vi "main.vi"() -> ()   [LabVIEW 2018]
panel:
  in  "stop":bool
  out "Numeric":i32
  out "A0":bool
  out "A1":bool
  out "A2":bool
  out "A4":bool
  in  "Count":bool
  in  "Load":bool
  in  "I0":bool
  in  "I1":bool
  in  "I2":bool
  in  "I3":bool
  out "Finish":bool
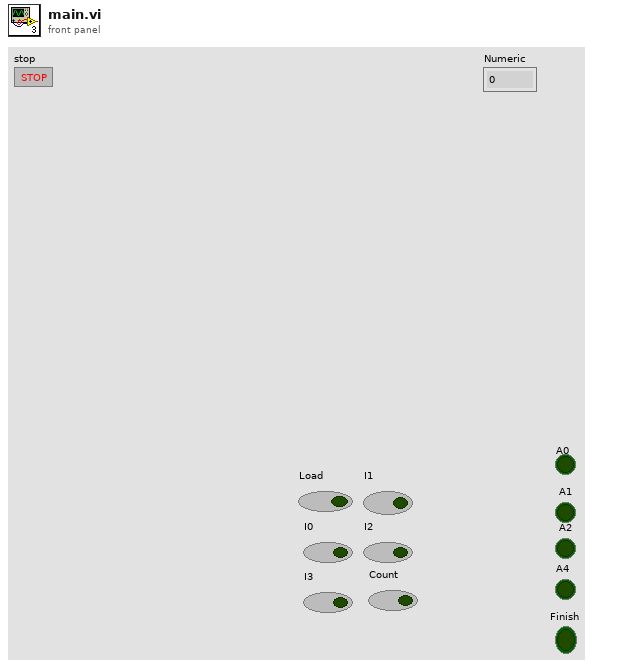
[diagram p1: front panel]
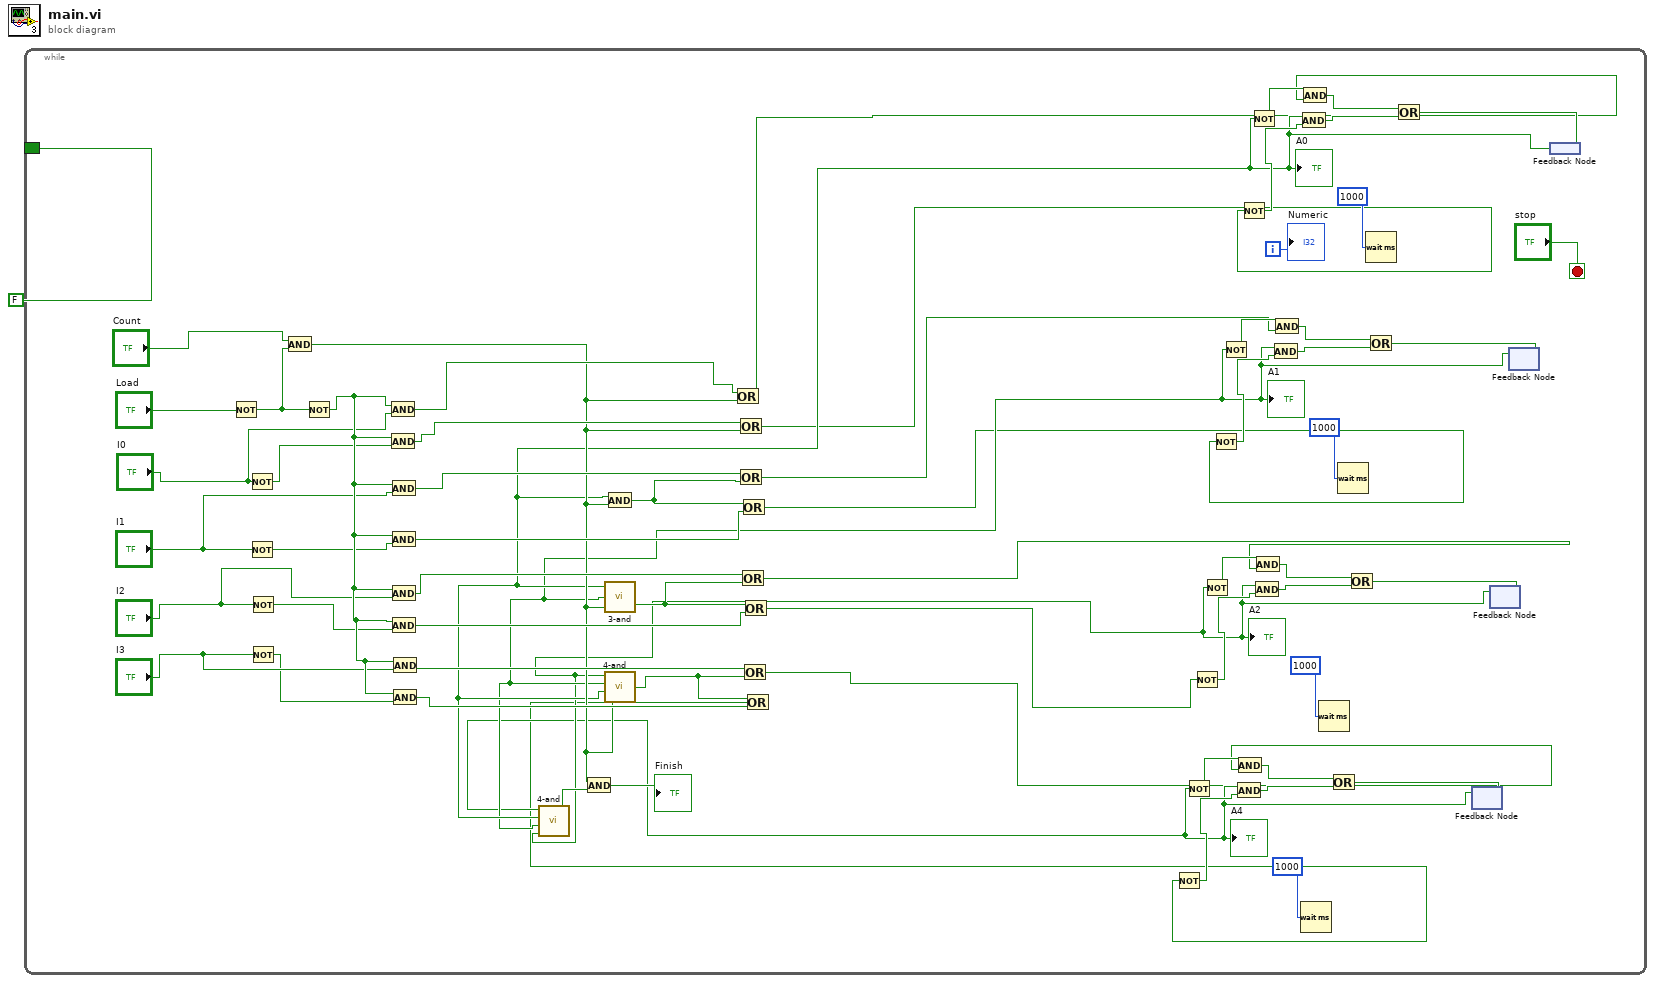
[diagram p0: block diagram]
diagram:
  n1 = while {
    border: FALSE -> [_]
    i -> [w63]
    stop <- "stop" stop-if-true
    n2 = Not(x="Load") -> (.not. x?=w37:bool)
    n3 = Not(x="I0") -> (.not. x?=w34:bool)
    n4 = Not(x="I1") -> (.not. x?=w32:bool)
    n5 = Not(x="I2") -> (.not. x?=w30:bool)
    n6 = Not(x="I3") -> (.not. x?=w28:bool)
    n7 = And(x="Count", y=w37) -> (x .and. y?=w16:bool)
    n8 = Not(x=w37) -> (.not. x?=w36:bool)
    n9 = And(x=w36, y="I0") -> (x .and. y?=w26:bool)
    n10 = And(x=w36, y=w34) -> (x .and. y?=w25:bool)
    n11 = And(x=w36, y="I1") -> (x .and. y?=w24:bool)
    n12 = And(x=w36, y=w32) -> (x .and. y?=w23:bool)
    n13 = And(x=w36, y="I2") -> (x .and. y?=w22:bool)
    n14 = And(x=w36, y=w30) -> (x .and. y?=w21:bool)
    n15 = And(x=w36, y="I3") -> (x .and. y?=w20:bool)
    n16 = And(x=w36, y=w28) -> (x .and. y?=w19:bool)
    n17 = Or(x=w26, y=w16) -> (x .or. y?=w12:bool)
    n18 = Or(x=w25, y=w16) -> (x .or. y?=w11:bool)
    n19 = Not(x=w11) -> (.not. x?=w58:bool)
    n20 = Wait (ms)(milliseconds to wait=u32 1000) -> ()  [unwired: 1 out]
    n21 = Wait (ms)(milliseconds to wait=u32 1000) -> ()  [unwired: 1 out]
    n22 = Wait (ms)(milliseconds to wait=u32 1000) -> ()  [unwired: 1 out]
    n23 = Wait (ms)(milliseconds to wait=u32 1000) -> ()  [unwired: 1 out]
    n24 = feedback #1() -> (w4:bool)  [unwired: 1 in]
    "A4" <- w4
    n25 = Not(x=w4) -> (.not. x?=w41:bool)
    n26 = feedback #2() -> (w7:bool)  [unwired: 1 in]
    "A2" <- w7
    n27 = Not(x=w7) -> (.not. x?=w47:bool)
    n28 = feedback #3() -> (w10:bool)  [unwired: 1 in]
    "A1" <- w10
    n29 = Not(x=w10) -> (.not. x?=w53:bool)
    n30 = feedback #4() -> (w13:bool)
    "A0" <- w13
    n31 = call "4-and.vi"("Boolean 4"=w7, "Boolean 3"=w10, "Boolean 2"=w13, "Boolean"=w4) -> ("Boolean 5"=w27:bool)
    n32 = And(x=w16, y=w27) -> (x .and. y?=→"Finish":bool)
    n33 = And(x=w13, y=w16) -> (x .and. y?=w18:bool)
    n34 = call "3-and.vi"("Boolean 2"=w16, "Boolean 4"=w10, "Boolean 3"=w13) -> ("Boolean"=w14:bool)
    n35 = call "4-and.vi"("Boolean 4"=w16, "Boolean 3"=w13, "Boolean 2"=w10, "Boolean"=w7) -> ("Boolean 5"=w17:bool)
    n36 = Or(x=w24, y=w18) -> (x .or. y?=w9:bool)
    n37 = Or(x=w22, y=w14) -> (x .or. y?=w6:bool)
    n38 = Or(x=w18, y=w23) -> (x .or. y?=w8:bool)
    n39 = Or(x=w20, y=w17) -> (x .or. y?=w3:bool)
    n40 = Or(x=w14, y=w21) -> (x .or. y?=w5:bool)
    n41 = Or(x=w17, y=w19) -> (x .or. y?=w2:bool)
    n42 = Not(x=w2) -> (.not. x?=w40:bool)
    n43 = Not(x=w5) -> (.not. x?=w46:bool)
    n44 = Not(x=w8) -> (.not. x?=w52:bool)
    n45 = And(x=w4, y=w40) -> (x .and. y?=w43:bool)
    n46 = And(x=w41, y=w3) -> (x .and. y?=w44:bool)
    n47 = Not(x=w13) -> (.not. x?=w59:bool)
    n48 = And(x=w7, y=w46) -> (x .and. y?=w49:bool)
    n49 = And(x=w47, y=w6) -> (x .and. y?=w50:bool)
    n50 = And(x=w10, y=w52) -> (x .and. y?=w55:bool)
    n51 = And(x=w53, y=w9) -> (x .and. y?=w56:bool)
    n52 = And(x=w13, y=w58) -> (x .and. y?=w61:bool)
    n53 = And(x=w59, y=w12) -> (x .and. y?=w62:bool)
    n54 = Or(x=w44, y=w43) -> (x .or. y?=w42:bool)
    n55 = Or(x=w50, y=w49) -> (x .or. y?=w48:bool)
    n56 = Or(x=w56, y=w55) -> (x .or. y?=w54:bool)
    n57 = Or(x=w62, y=w61) -> (x .or. y?=w60:bool)
    n58 = feedback-in #1(w42) -> ()
    n59 = feedback-in #2(w48) -> ()
    n60 = feedback-in #3(w54) -> ()
    n61 = feedback-in #4(w60) -> ()
    "Numeric" <- w63
  }
